vi "Actor Core.vi"(8 "error in":errorcluster, 11 "Phoenix in":refnum<class "Phoenix.lvclass">) -> (0 "error out":errorcluster, 3 "Actor out":refnum<class "Actor.lvclass">)   [LabVIEW 2022 SP3, in "Phoenix.lvlib" / "Phoenix.lvclass"]
doc: "(<B>Filename</B>: Actor Framework.lvlib:Actor.lvclass:Actor Core.vi)\n\nReceives messages to the actor, reacts to them, and initiates any error handling that may shut the actor down.\n\nDescendant classes may override this VI to append parallel tasks for the actor to complete while it handles messages. Overrides use the Call Parent Class Method node."
uses:
  Phoenix.lvclass
  C:/Program Files (x86)/National Instruments/LabVIEW 2022/vi.lib/ActorFramework/Actor/Actor.lvclass
  <vilib>/ActorFramework/Actor/Actor.lvclass
  UDP Input.ctl
  Vision/Vision/Vision.lvclass
  Phoenix.lvclass/Phoenix.ctl
  <vilib>/ActorFramework/Actor/Actor.lvclass/Actor.ctl
  <vilib>/ActorFramework/Message Enqueuer/Message Enqueuer.lvclass/Message Enqueuer.ctl
  UDP Data Receiver/UDP Data Receiver Messages/Start Receiving Msg/Start Receiving Msg.lvclass/Start Receiving Msg.ctl
  <vilib>/ActorFramework/Message Enqueuer/Init from Existing Queue.vi
  <vilib>/ActorFramework/Message Enqueuer/Enqueue.vi
  UDP Data Receiver/UDP Data Receiver Messages/Stop Receiving Msg/Stop Receiving Msg.lvclass
  C:/Program Files (x86)/National Instruments/LabVIEW 2022/vi.lib/ActorFramework/Message/Message.lvclass
  <vilib>/ActorFramework/Stop Msg/Stop Msg.lvclass
  UDP Data Receiver/UDP Data Receiver Messages/Start Receiving Msg/Start Receiving Msg.lvclass
  <vilib>/ActorFramework/Message Priority Queue/Priority Enqueue.vi
  <vilib>/ActorFramework/Message Enqueuer/Message Enqueuer.lvclass
  <vilib>/MGI/Monitored Actor/Monitored Actor/Monitored Actor/Monitored Actor.lvclass
panel:
  in  "Vision ON/OFF":bool
  out "Field Drawing":picture
  in  "Vision RX Counter":timestamp
  out "FPS":dbl
  out "RX":bool
  in  "Stop":bool
  in  "Vision Input":T1={"Local IP"="", "Port"="10020", "Server IP"="224.5.23.2"}
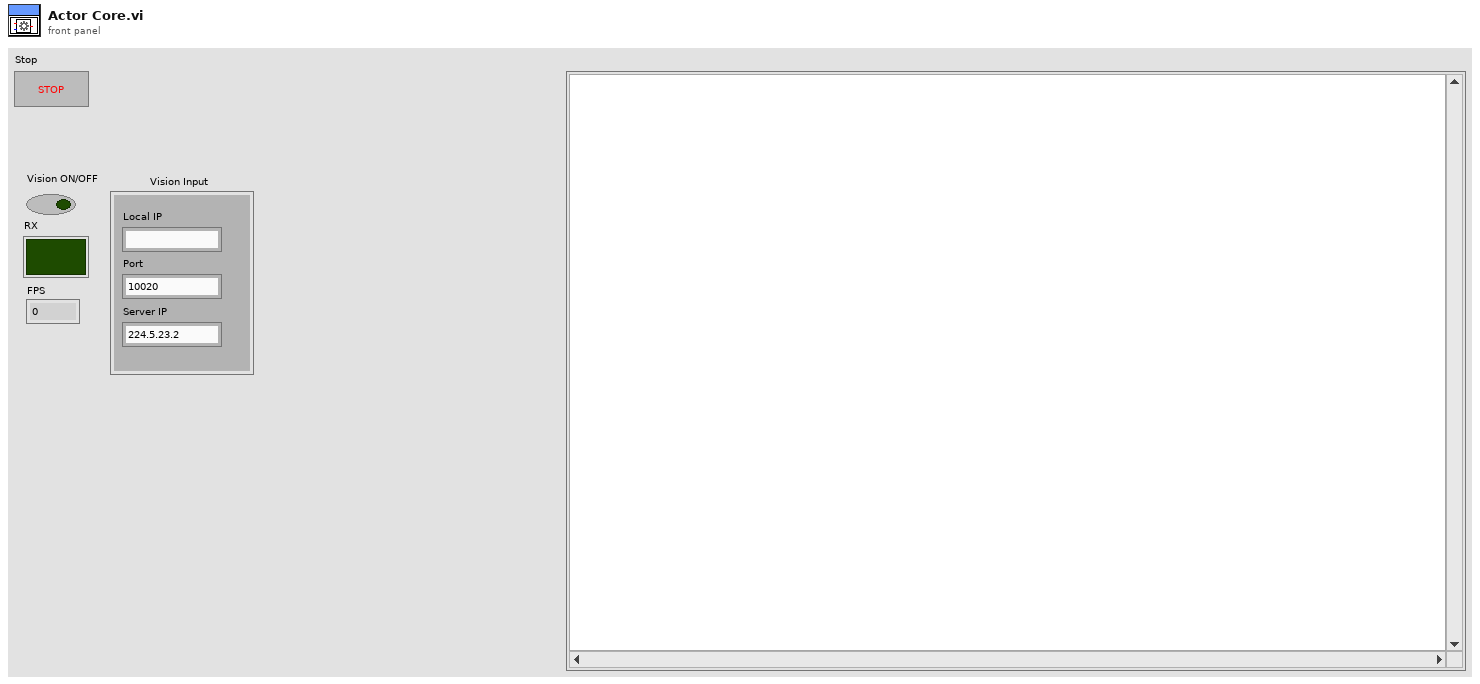
[diagram p1: front panel]
types:
  T1 = typedef "UDP Input.ctl" = cluster{"Local IP":string, "Port":string, "Server IP":string}
  T2 = cluster{"Vision RX":refnum<user-event>, "Stop":refnum<user-event>}
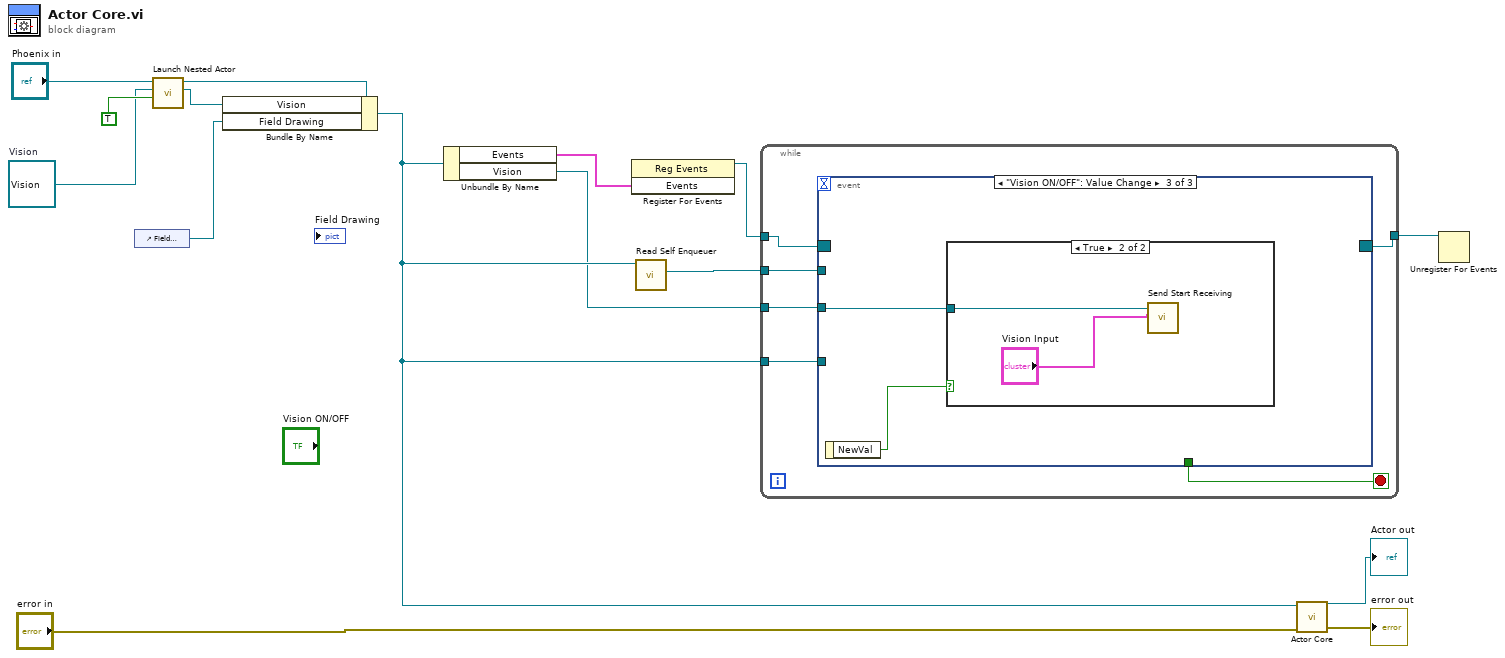
[diagram p0: block diagram]
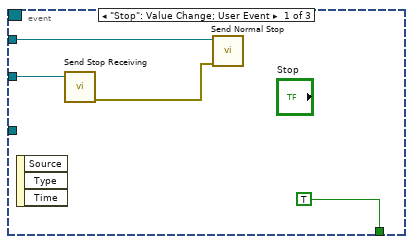
[diagram p2: hidden frame]
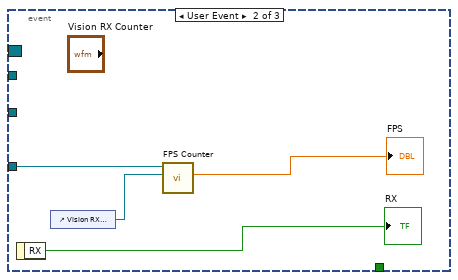
[diagram p3: hidden frame]
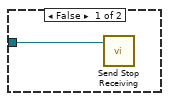
[diagram p4: hidden frame]
diagram:
  w2 = refnum<class "Vision.lvclass"> refnum  # Vision
  n1 = control-ref of="Field Drawing"() -> (w1:refnum<vi>)
  n2 = call <vilib>:"Launch Nested Actor.vi"("Auto-stop? (T)"=TRUE, "Nested Actor"=w2, "Caller Actor in"="Phoenix in") -> ("Nested Actor's Enqueuer"=w5:refnum<class "Message Enqueuer.lvclass">, "Caller Actor out"=w6:refnum<class "Phoenix.lvclass">)  [unwired: 6 in, 1 out]
  n3 = Bundle By Name(cluster=w6, "Vision"=w5, "Field Drawing"=w1) -> (w4:refnum<class "Phoenix.lvclass">)
  n4 = Unbundle By Name(w4) -> ("Events"=w12:T2, "Vision"=w3:refnum<class "Message Enqueuer.lvclass">)
  n5 = register-events(w12) -> (reference out=w11:refnum<event-registration>)  [unwired: 2 in, 1 out]
  n6 = call <vilib>:"Read Self Enqueuer.vi"("Actor"=w4) -> ("Self Enqueuer"=w9:refnum<class "Message Enqueuer.lvclass">)  [unwired: 10 in]
  n7 = while {
    tunnel: w11 -> [w20]
    tunnel: [w19] -> w10
    tunnel: w9 -> [w18]
    tunnel: w4 -> [w17]
    tunnel: w3 -> [w16]
    stop <- w21 stop-if-true
    n8 = event shown="[2] \"Vision ON/OFF\": Value Change" {
      selector: w20 -> [_ _ _]
      dyn-events: [_ _ _] -> w19
      timeout: _ -> [_ _ _]
      tunnel: [TRUE _ _] -> w21
      tunnel: w18 -> [w24 _ _]
      tunnel: w17 -> [_ w26 _]
      tunnel: w16 -> [w23 _ w31]
      event "Stop": Value Change; User Event {
        n9 = event-data() -> ()  [unwired: 1 in, 3 out]
        n10 = call "Send Stop Receiving.vi"("Message Enqueuer"=w23) -> ("error out"=w22:errorcluster)  [unwired: 9 in, 1 out]
        n11 = call <vilib>:"Send Normal Stop.vi"("error in (no error)"=w22, "Message Enqueuer"=w24) -> ()  [unwired: 9 in, 1 out]
      }
      event User Event {
        n12 = event-data() -> ("RX"=→"RX":bool)  [unwired: 1 in]
        n13 = control-ref of="Vision RX Counter"() -> (w28:refnum<vi>)
        n14 = call-dynamic "FPS Counter.vi"("Counter Reference"=w28, "Phoenix in"=w26) -> ("FPS"=→"FPS":dbl)  [unwired: 7 in, 2 out]
      }
      event "Vision ON/OFF": Value Change {
        n15 = event-data() -> ("NewVal"=w30:bool)  [unwired: 1 in]
        n16 = case shown="True" w30 {
          tunnel: w31 -> [w32 w34]
          frame False {
            n17 = call "Send Stop Receiving.vi"("Message Enqueuer"=w32) -> ()  [unwired: 9 in, 2 out]
          }
          frame True {
            n18 = call "Send Start Receiving.vi"("Input"="Vision Input", "Message Enqueuer"=w34) -> ()  [unwired: 8 in, 2 out]
          }
        }
      }
    }
  }
  n19 = call-parent "Actor Core.vi"("error in"="error in", "Actor in"=w4) -> ("error out"=→"error out":errorcluster, "Actor out"=→"Actor out":refnum<class "Actor.lvclass">)  [unwired: 8 in]
  n20 = Unregister For Events(event registration refnum=w10) -> ()  [unwired: 1 in, 1 out]
